vi "send_to_labbook.vi"(6 "File":path, 8 "Text":string="Print", 9 "author":string="Print", 10 "Title":string="Print", 11 "logbook name":string="AS3elog") -> (3 "Answer":string)   [LabVIEW 2013]
uses:
  <vilib>/httpClient/MultipartData.ctl
  <vilib>/httpClient/LabVIEWHTTPClient.lvlib
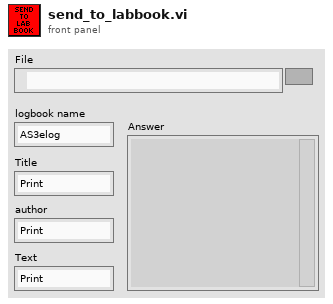
[diagram p1: front panel]
types:
  T1 = typedef "LabVIEWHTTPClient.lvlib/MultipartData.ctl" = cluster{"Name":string, "Value":string, "File":path, "Filename":string, "MIME type":string}
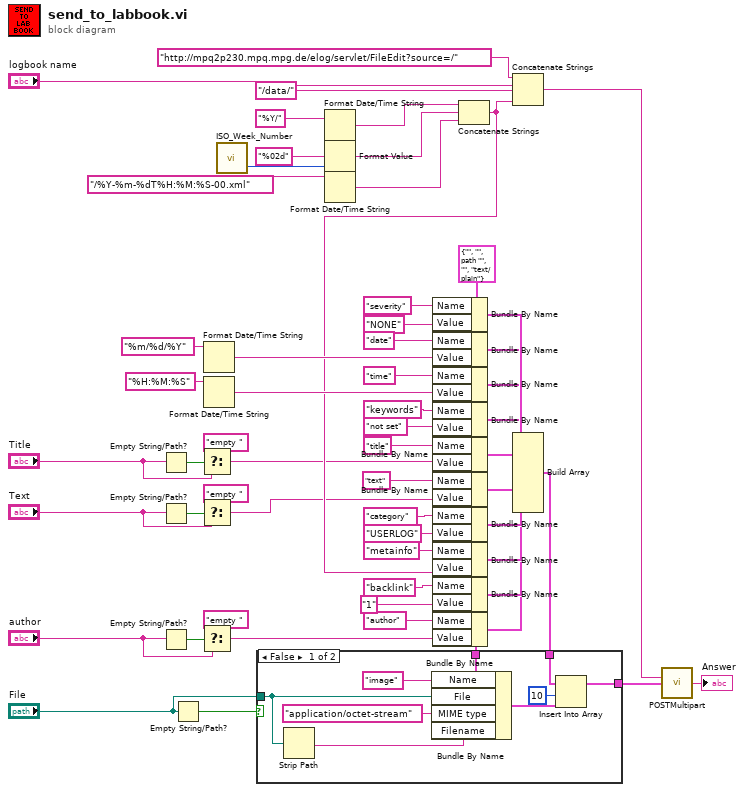
[diagram p0: block diagram]
diagram:
  w14 = T1 {"Name"="", "Value"="", "File"=path "", "Filename"="", "MIME type"="text/plain"} ("Element")
  n1 = Empty String/Path?(string/path="Title") -> (empty?=w22:bool)
  n2 = Empty String/Path?(string/path="Text") -> (empty?=w18:bool)
  n3 = Empty String/Path?(string/path="author") -> (empty?=w13:bool)
  n4 = Empty String/Path?(string/path="File") -> (empty?=w1:bool)
  n5 = Select(t="empty ", s=w22, f="Title") -> (s? t:f=w19:string)
  n6 = Select(t="empty ", s=w18, f="Text") -> (s? t:f=w16:string)
  n7 = Select(t="empty ", s=w13, f="author") -> (s? t:f=w10:string)
  n8 = Format Date/Time String(time format string (%c)="%m/%d/%Y") -> (date/time string=w45:string)  [unwired: 2 in]
  n9 = Format Date/Time String(time format string (%c)="%H:%M:%S") -> (date/time string=w37:string)  [unwired: 2 in]
  n10 = call "ISO_Week_Number.vi"() -> ("ISO week"=w39:i32)  [unwired: 1 in, 1 out]
  n11 = Format Date/Time String(time format string (%c)="%Y/") -> (date/time string=w43:string)  [unwired: 2 in]
  n12 = Format Value(format string="%02d", value (0)=w39) -> (output string=w40:string)  [unwired: 1 in]
  n13 = Format Date/Time String(time format string (%c)="/%Y-%m-%dT%H:%M:%S-00.xml") -> (date/time string=w41:string)  [unwired: 2 in]
  n14 = Bundle By Name(cluster=w14, "Name"="severity", "Value"="NONE") -> (w32:T1)
  n15 = Bundle By Name(cluster=w14, "Name"="date", "Value"=w45) -> (w31:T1)
  n16 = Bundle By Name(cluster=w14, "Name"="time", "Value"=w37) -> (w30:T1)
  n17 = Bundle By Name(cluster=w14, "Name"="keywords", "Value"="not set") -> (w29:T1)
  n18 = Bundle By Name(cluster=w14, "Name"="title", "Value"=w19) -> (w28:T1)
  n19 = Bundle By Name(cluster=w14, "Name"="text", "Value"=w16) -> (w27:T1)
  n20 = Bundle By Name(cluster=w14, "Name"="category", "Value"="USERLOG") -> (w26:T1)
  n21 = Bundle By Name(cluster=w14, "Name"="backlink", "Value"="1") -> (w24:T1)
  n22 = Bundle By Name(cluster=w14, "Name"="author", "Value"=w10) -> (w9:T1)
  n23 = Concatenate Strings(w43, w40, w41) -> (w23:string)
  n24 = Bundle By Name(cluster=w14, "Name"="metainfo", "Value"=w23) -> (w25:T1)
  n25 = Concatenate Strings("http://mpq2p230.mpq.mpg.de/elog/servlet/FileEdit?source=/" ("string"), "logbook name", "/data/" ("string"), w23) -> (w33:string)
  n26 = Build Array(w32, w31, w30, w29, w28, w27, w26, w25, w24, w9) -> (w2:T1[])
  n27 = case shown="False" w1 {
    tunnel: w14 -> [w64 _]
    tunnel: "File" -> [w63 _]
    tunnel: [w62 w68] -> w3
    tunnel: w2 -> [w61 w68]
    frame False {
      n28 = Strip Path(path=w63) -> (name=w65:string)  [unwired: 1 out]
      n29 = Bundle By Name(cluster=w64, "Name"="image", "File"=w63, "MIME type"="application/octet-stream", "Filename"=w65) -> (w60:T1)
      n30 = Insert Into Array(array=w61, index=10, new element=w60) -> (w62:T1[])
    }
    frame True {
    }
  }
  n31 = call <vilib>:"POSTMultipart.vi"("url"=w33, "data"=w3) -> ("body"=→"Answer":string)  [unwired: 10 in, 3 out]
